vi "test - csm dependencies.vi"(8 "error in (no error)":errorcluster, 11 "TestCase in":refnum<class "testcase-miscellaneous.lvclass">) -> (0 "error out":errorcluster, 3 "TestCase out":refnum<class "testcase-miscellaneous.lvclass">)   [LabVIEW 2017, in "testcase-miscellaneous.lvclass"]
uses:
  testcase-miscellaneous.lvclass
  <vilib>/addons/_JKI Toolkits/VI Tester/TestCase.llb/TestCase.lvclass
  src/user.lib/_NEVSTOP/Communicable State Machine(CSM)/Communicable State Machine.lvlib
  src/user.lib/_NEVSTOP/Communicable State Machine(CSM)/_Shared/CSM Shared.lvlib
  C:/Program Files (x86)/National Instruments/LabVIEW 2017/vi.lib/addons/_JKI Toolkits/VI Tester/TestCase.llb/TestCase.lvclass
panel:
  out "Dependency Paths":path[](array[path])
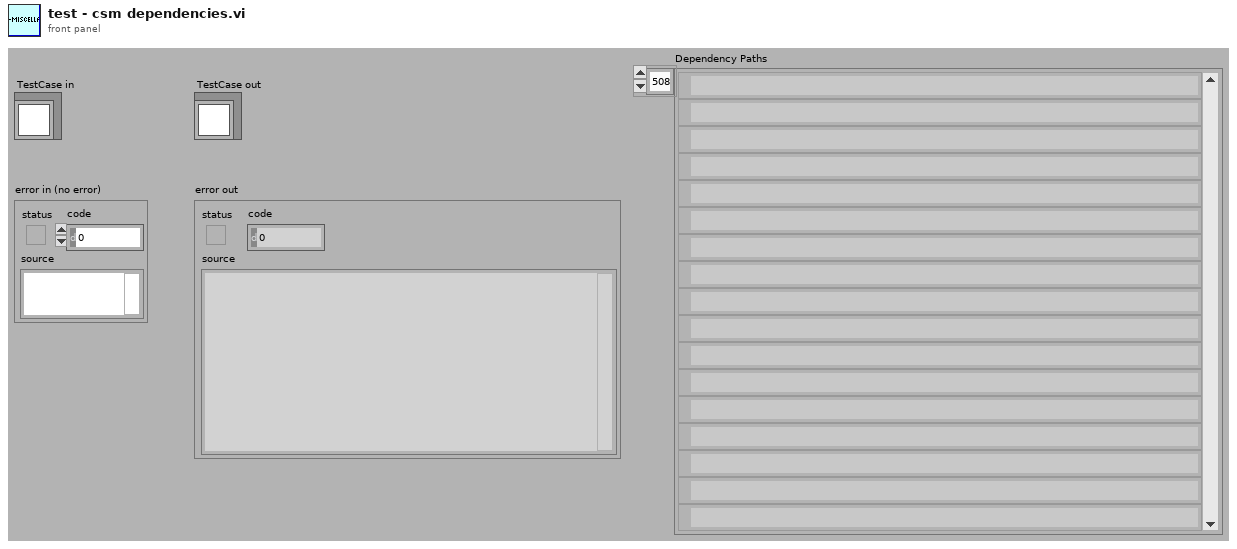
[diagram p1: front panel]
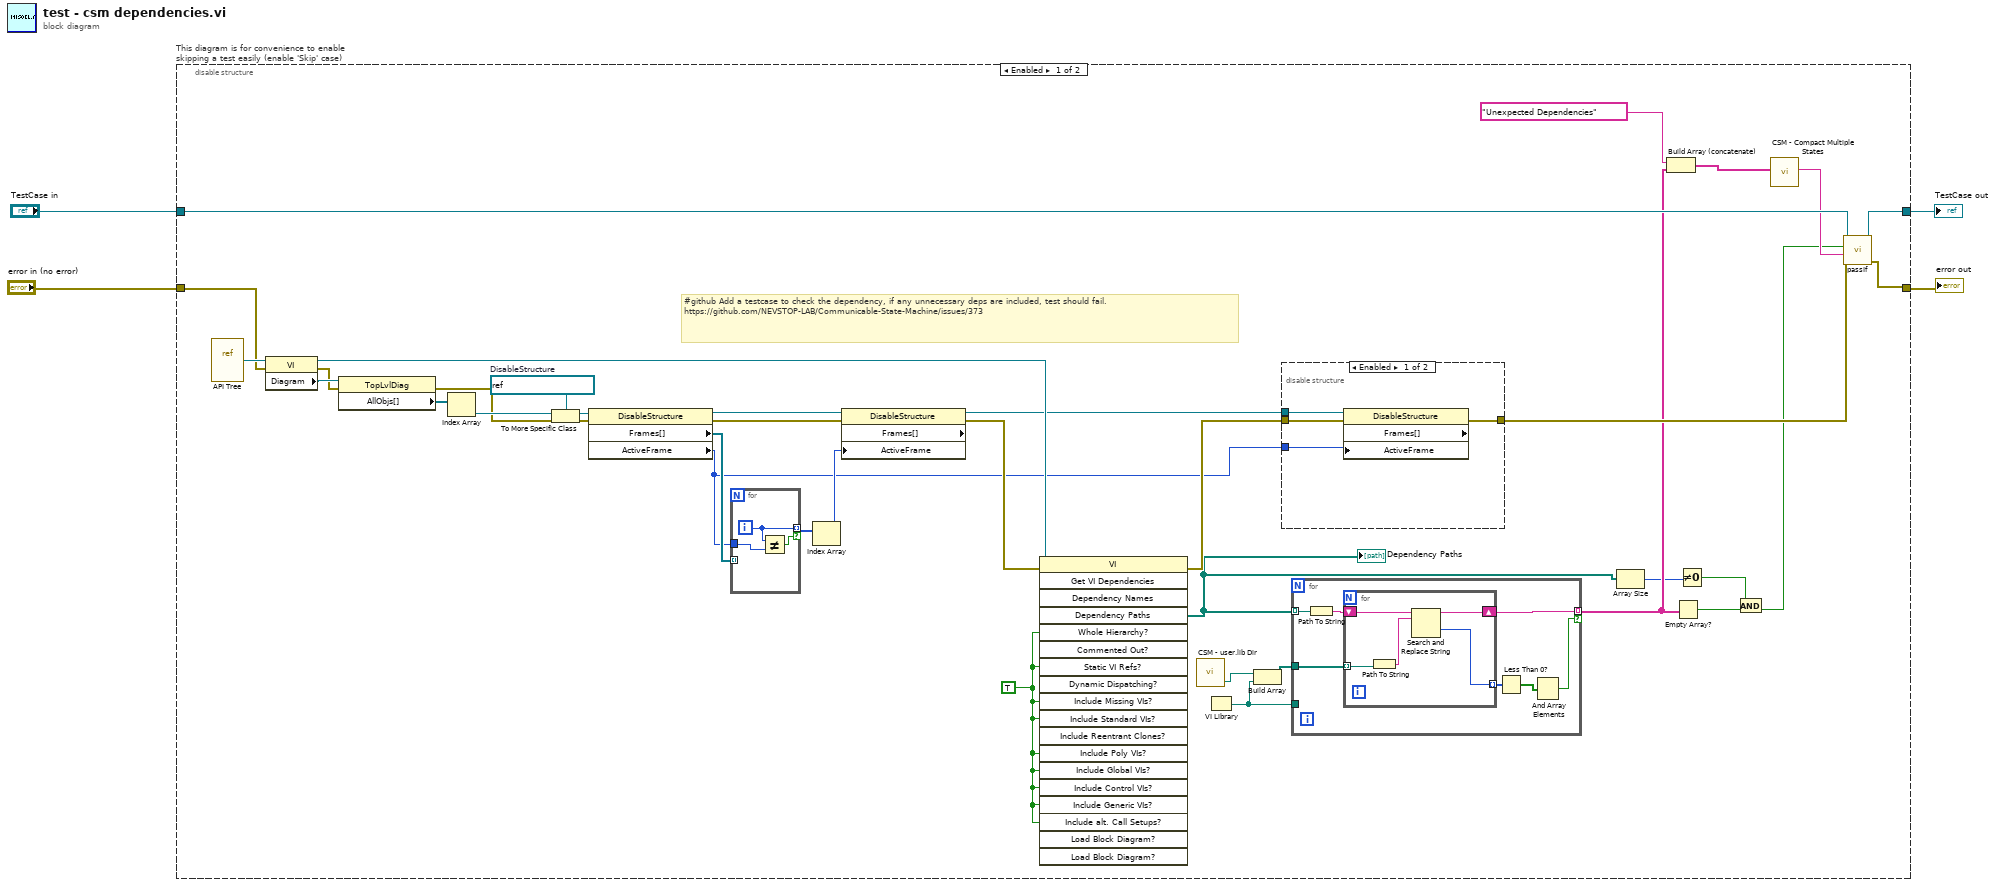
[diagram p0: block diagram]
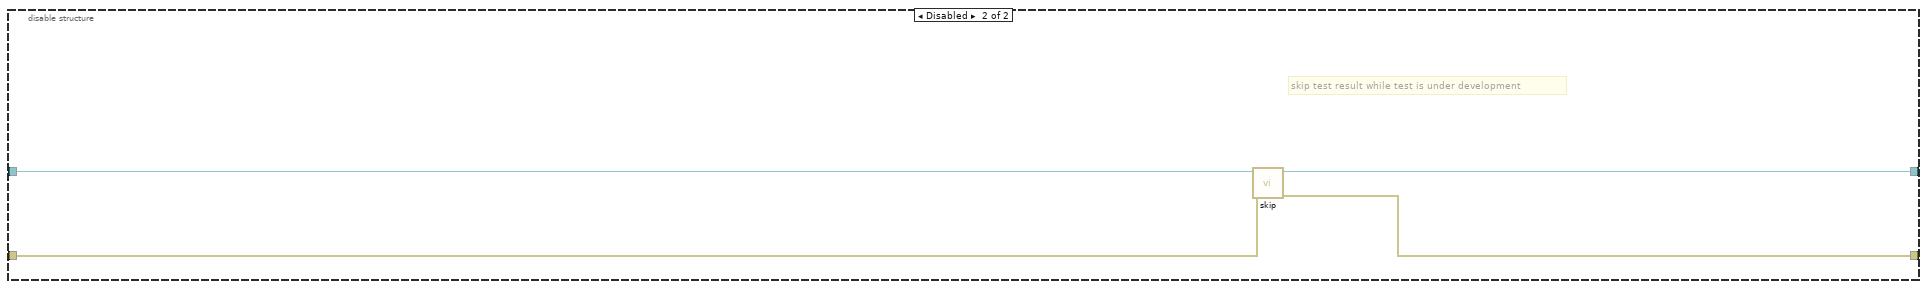
[diagram p3: hidden frame]
diagram:
  n1 = disable-structure "This diagram is for convenience to enable skipping a test easily (enable 'Skip' case)" shown="Enabled" {
    disable-tunnel: "TestCase in" -> [w41 w65]
    disable-tunnel: [w40 w63] -> w1
    disable-tunnel: [w39 w64] -> w3
    disable-tunnel: "error in (no error)" -> [w17 w62]
    frame Enabled {
      w29 = refnum<vi> refnum  # DisableStructure
      w34 = TRUE ("Include Missing Items?")
      # "#github Add a testcase to check the dependency, if any unnecessary deps are included, test should fail. \nhttps://github.com/NEVSTOP-LAB/Communicable-State-Machine/issues/373"
      n2 = vi-ref "API Tree.vi"() -> (w36:refnum<vi>)
      n3 = property class="VI"(reference=w36, error in=w17) -> (reference out=w33:refnum<vi>, error out=w16:errorcluster, "Diagram"=w32:refnum<vi>)
      n4 = property class="TopLvlDiag"(reference=w32, error in=w16) -> (error out=w15:errorcluster, "AllObjs[]"=w31:refnum<vi>[])  [unwired: 1 out]
      n5 = Index Array(array=w31) -> (element=w30:refnum<vi>)  [unwired: 1 in]
      n6 = To More Specific Class(target class=w29, reference=w30, error in=w15) -> (specific class reference=w27:refnum<vi>, error out=w28:errorcluster)
      n7 = property class="DisableStructure"(reference=w27, error in=w28) -> (reference out=w26:refnum<vi>, error out=w25:errorcluster, "Frames[]"=w24:refnum<vi>[], "ActiveFrame"=w18:i16)
      n8 = for {
        tunnel: w24 -> [_] mode=indexing
        tunnel: [w61] -> w23 mode=indexing if=w59
        tunnel: w18 -> [w60]
        i -> [w61]
        n9 = Not Equal?(x=w61, y=w60) -> (x != y?=w59:bool)
      }
      n10 = Index Array(array=w23) -> (element=w22:i32)  [unwired: 1 in]
      n11 = property class="DisableStructure" props=["Frames[]", "ActiveFrame"](reference=w26, error in=w25, "ActiveFrame"=w22) -> (reference out=w20:refnum<vi>, error out=w21:errorcluster)  [unwired: 1 out]
      n12 = invoke class="VI" method="Get VI Dependencies"(reference=w33, error in=w21, "Whole Hierarchy?"=w34, "Static VI Refs?"=w34, "Include Missing VIs?"=w34, "Include Standard VIs?"=w34, "Include Poly VIs?"=w34, "Include Global VIs?"=w34, "Include Control VIs?"=w34, "Include Generic VIs?"=w34, "Include alt. Call Setups?"=w34) -> (error out=w19:errorcluster, "Dependency Paths"=w9:path[])  [unwired: 8 in, 17 out]
      "Dependency Paths" <- w9
      n13 = call "CSM - user.lib Dir.vi"() -> ("<LabVIEW>"=w6:path)  [unwired: 2 in, 1 out]
      n14 = VI Library() -> (path=w5:path)
      n15 = Build Array(w6, w5) -> (w7:path[])
      n16 = disable-structure shown="Enabled" {
        disable-tunnel: w20 -> [w57 _]
        disable-tunnel: w19 -> [w56 w58]
        disable-tunnel: w18 -> [w55 _]
        disable-tunnel: [w54 w58] -> w14
        frame Enabled {
          n17 = property class="DisableStructure" props=["Frames[]", "ActiveFrame"](reference=w57, error in=w56, "ActiveFrame"=w55) -> (error out=w54:errorcluster)  [unwired: 2 out]
        }
        frame Disabled {
        }
      }
      n18 = for {
        tunnel: w9 -> [w48] mode=indexing
        tunnel: w7 -> [w46]
        tunnel: [w44] -> w13 mode=indexing if=w42
        tunnel: w5 -> [_]
        n19 = Path To String(path=w48) -> (string=w47:string)
        n20 = for {
          tunnel: w46 -> [w52] mode=indexing
          tunnel: [w50] -> w45 mode=indexing
          shift-right: [w49] -> w44
          shift-left: w47 -> [w53]
          n21 = Path To String(path=w52) -> (string=w51:string)
          n22 = Search and Replace String(input string=w53, search string=w51) -> (result string=w49:string, offset past replacement=w50:i32)  [unwired: 6 in, 2 out]
        }
        n23 = Less Than 0?(x=w45) -> (x < 0?=w43:bool[])
        n24 = And Array Elements(Boolean array=w43) -> (logical AND=w42:bool)
      }
      n25 = Array Size(array=w9) -> (size(s)=w10:i32)
      n26 = Build Array (concatenate)("Unexpected Dependencies" ("message (\"\")"), w13) -> (w38:string[])
      n27 = Empty Array?(array=w13) -> (empty?=w8:bool)
      n28 = Not Equal To 0?(x=w10) -> (x != 0?=w11:bool)
      n29 = And(x=w11, y=w8) -> (x .and. y?=w12:bool)
      n30 = call "CSM - Compact Multiple States.vi"("Multiple States"=w38) -> ("States"=w37:string)  [unwired: 9 in]
      n31 = call-dynamic "passIf.vi"("error in (no error)"=w14, "message (\"\")"=w37, "pass"=w12, "TestCase in"=w41) -> ("error out"=w39:errorcluster, "TestCase out"=w40:refnum<class "testcase-miscellaneous.lvclass">)  [unwired: 6 in]
    }
    frame Disabled {
      # "skip test result while test is under development"
      n32 = call <vilib>:"skip.vi"("error in (no error)"=w62, "TestCase in"=w65) -> ("error out"=w64:errorcluster, "TestCase out"=w63:refnum<class "testcase-miscellaneous.lvclass">)  [unwired: 8 in]
    }
  }
  "error out" <- w3
  "TestCase out" <- w1
